vi "diffAndFilter.vi"(2 "data":waveform(dbl)[](array[waveform])) -> (0 "error out":errorcluster, 1 "d/dt":dynamicdata(graph) caption="Filtered Signal")   [LabVIEW 2018]
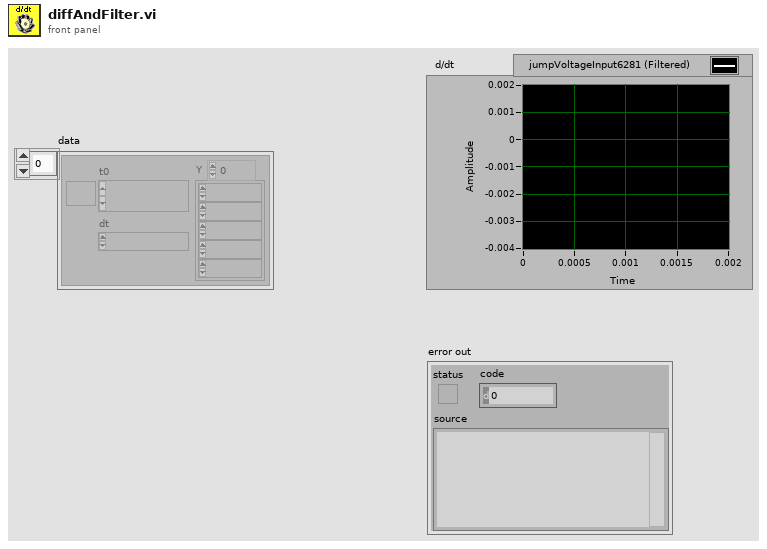
[diagram p1: front panel]
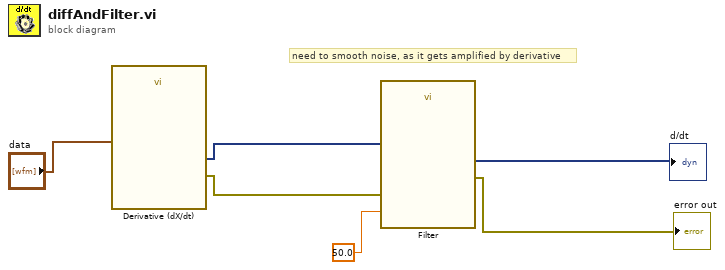
[diagram p0: block diagram]
diagram:
  # "need to smooth noise, as it gets amplified by derivative"
  n1 = call "Derivative (dX/dt)"("Signals"="data") -> ("error out"=w4:errorcluster, "Result"=w6:dynamicdata)  [unwired: 5 in]
  n2 = call "Filter"("error in (no error)"=w4, "Lower Cut-Off"=50.0, "Signal"=w6) -> ("error out"=→"error out":errorcluster, "Filtered Signal"=→"d/dt":dynamicdata)  [unwired: 7 in]
